vi "Test QR Code Memory Allocation.vi"(11 "Test Case In":refnum<class "02_FeatureDetection.lvclass">) -> (0 "error out":errorcluster, 3 "Test Case Out":refnum<class "02_FeatureDetection.lvclass">)   [LabVIEW 2020, in "test.lvlib" / "02_FeatureDetection.lvclass"]
uses:
  02_FeatureDetection.lvclass
  usr/local/natinst/LabVIEW-2024-64/vi.lib/Astemes/LUnit/Test Case.lvclass
  feature_detection/WeChat QR Code Detector/Detection.ctl
  common/Image Points Quad (Float).ctl
  common/Image Point (Float).ctl
  common/Image Size (Integer).ctl
  feature_detection/QR Code Encoder/Correction Levels.ctl
  feature_detection/QR Code Encoder/QR Code Encoder.lvclass/QR Code Encoder.ctl
  feature_detection/WeChat QR Code Detector/WeChat QR Code Detector.lvclass/WeChat QR Code Detector.ctl
  <vilib>/Astemes/LUnit/Test Case.lvclass/Test Case.ctl
  feature_detection/QR Code Encoder/Create (Structured Append).vi
  image/New Image (Greyscale Preallocated).vi
  image/New Image (Greyscale Array).vi
  image/Draw Image to Picture (Greyscale).vi
  feature_detection/WeChat QR Code Detector/Detect and Decode Multiple (Greyscale).vi
  feature_detection/QR Code Encoder/CreateCore.vi
  image/New Image (Greyscale Preallocated).vi/6598b9e0-8a08-46f5-91fd-ca1b87217137.vi
  image/Draw Image to Picture (Greyscale).vi/9ae995ca-ccda-485c-89ac-02736fde3e8e.vi
  feature_detection/WeChat QR Code Detector/Detect and Decode Multiple (Greyscale).vi/de44e2b3-a41c-416e-9770-09f180cbffa1.vi
  <vilib>/Astemes/LUnit/Append Pass Result.vi
  <vilib>/Astemes/LUnit/Append Fail Result.vi
  <vilib>/Astemes/LUnit/Run In UI.vi
  <vilib>/Utility/error.llb/Clear Errors.vi
  <vilib>/Utility/error.llb/Error Cluster From Error Code.vi
  feature_detection/QR Code Encoder/Encode (Structured Append).vi
  feature_detection/WeChat QR Code Detector/Create (Model Files Folder).vi
  feature_detection/QR Code Encoder/QR Code Encoder.lvclass
  feature_detection/WeChat QR Code Detector/WeChat QR Code Detector.lvclass
  image/image.lvlib
  <vilib>/Astemes/LUnit/Test Case.lvclass
  common/common.lvlib
panel:
  out "Picture":picture
  out "Array":cluster{"Detections":T1[]}[](array[cluster])
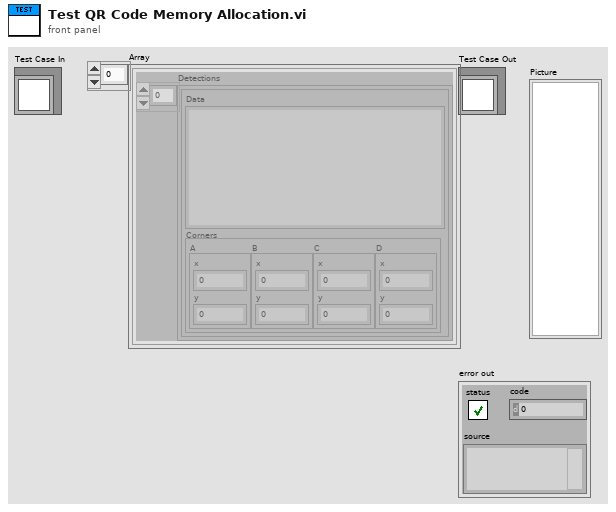
[diagram p1: front panel]
types:
  T1 = typedef "feature_detection.lvlib/WeChat QR Code Detector.lvclass/Detection.ctl" = cluster{"Data":string, "Corners":T2}
  T2 = typedef "common.lvlib/Image Points Quad (Float).ctl" = cluster{"A":T3, "B":T3, "C":T3, "D":T3}
  T3 = typedef "common.lvlib/Image Point (Float).ctl" = cluster{"x":dbl, "y":dbl}
  T4 = typedef "feature_detection.lvlib/QR Code Encoder.lvclass/Correction Levels.ctl" = enum16{"Level L", "Level M", "Level Q", "Level H"}
  T5 = typedef "common.lvlib/Image Size (Integer).ctl" = cluster{"Width":u16, "Height":u16}
  T6 = typedef "image.lvlib/Greyscale Image.ctl" = refnum<data-value>
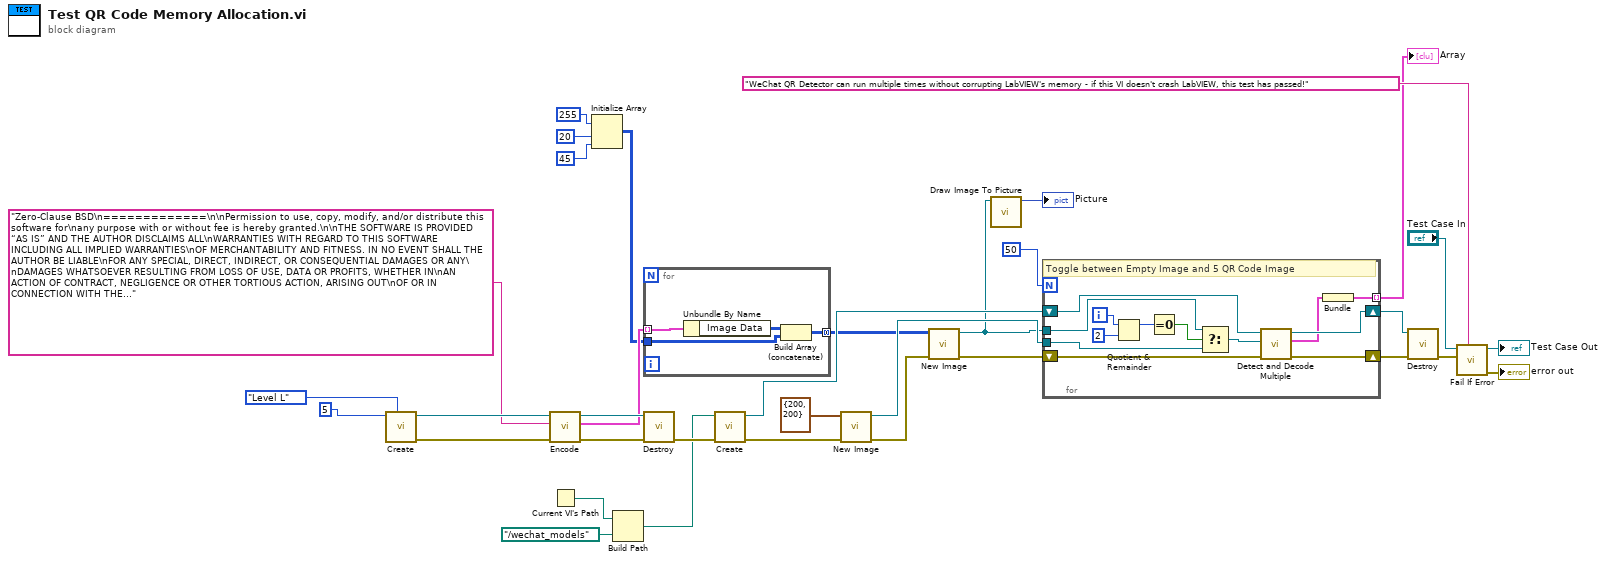
[diagram p0: block diagram]
diagram:
  n1 = call-poly "Create.vi"("Correction Level (Default: Level L)"=Correction_Levels."Level L", "Number of Structures"=u8 5) -> ("error out"=w18:errorcluster, "QR Code Encoder"=w20:refnum<class "QR Code Encoder.lvclass">)  [unwired: 8 in]
  n2 = call-poly "Encode.vi"("error in (no error)"=w18, "Data"="Zero-Clause BSD\n=============\n\nPermission to use, copy, modify, and/or distribute this software for\nany purpose with or without fee is hereby granted.\n\nTHE SOFTWARE IS PROVIDED “AS IS” AND THE AUTHOR DISCLAIMS ALL\nWARRANTIES WITH REGARD TO THIS SOFTWARE INCLUDING ALL IMPLIED WARRANTIES\nOF MERCHANTABILITY AND FITNESS. IN NO EVENT SHALL THE AUTHOR BE LIABLE\nFOR ANY SPECIAL, DIRECT, INDIRECT, OR CONSEQUENTIAL DAMAGES OR ANY\nDAMAGES WHATSOEVER RESULTING FROM LOSS OF USE, DATA OR PROFITS, WHETHER IN\nAN ACTION OF CONTRACT, NEGLIGENCE OR OTHER TORTIOUS ACTION, ARISING OUT\nOF OR IN CONNECTION WITH THE USE OR PERFORMANCE OF THIS SOFTWARE.", "QR Code Encoder in"=w20) -> ("error out"=w17:errorcluster, "QR Codes"=w9:cluster{"Image Data":u8[][]}[], "QR Code Encoder"=w19:refnum<class "QR Code Encoder.lvclass">)  [unwired: 6 in]
  n3 = Current VI's Path() -> (path=w3:path)
  n4 = Initialize Array(u8 255 ("element"), 20 ("dimension size"), 45 ("dimension size")) -> (w7:u8[][])
  n5 = Build Path(base path=w3, name or relative path=path "../wechat_models") -> (appended path=w2:path)
  n6 = for {
    tunnel: [w37] -> w14 mode=concatenating
    tunnel: w9 -> [w38] mode=indexing
    tunnel: w7 -> [w36]
    n7 = Unbundle By Name(w38) -> ("Image Data"=w35:u8[][])
    n8 = Build Array (concatenate)(w35, w36) -> (w37:u8[][])
  }
  n9 = call "Destroy.vi"("error in (no error)"=w17, "QR Code Encoder in"=w19) -> ("error out"=w15:errorcluster)  [unwired: 9 in]
  n10 = call-poly "Create.vi"("error in (no error)"=w15, "Model Files Directory"=w2) -> ("error out"=w30:errorcluster, "WeChat QR Code Detector"=w33:refnum<class "WeChat QR Code Detector.lvclass">)  [unwired: 8 in]
  n11 = call-poly "New Image.vi"("error in (no error)"=w30, "Preallocated Image Size (Default 0,0)"=T5 {"Width"=200, "Height"=200} ("Preallocated Image Size (Default: 0,0)")) -> ("error out"=w32:errorcluster, "Greyscale Image"=w31:T6)  [unwired: 8 in]
  n12 = call-poly "New Image.vi"("error in (no error)"=w32, "U8 Greyscale Data"=w14) -> ("error out"=w34:errorcluster, "Greyscale Image"=w13:T6)  [unwired: 8 in]
  n13 = call-poly "Draw Image To Picture.vi"("Greyscale Image Source in"=w13) -> ("Picture"=→"Picture":picture)  [unwired: 9 in, 1 out]
  n14 = for {
    N: 50 -> [_]
    tunnel: w13 -> [w45]
    tunnel: w31 -> [w44]
    shift-right: [w42] -> w29
    shift-left: w33 -> [w50]
    shift-right: [w41] -> w23
    shift-left: w34 -> [w51]
    tunnel: [w39] -> w21 mode=indexing
    i -> [w49]
    # "Toggle between Empty Image and 5 QR Code Image"
    n15 = Quotient & Remainder(x=w49, y=2) -> (x-y*floor(x/y)=w47:i32)  [unwired: 1 out]
    n16 = Equal To 0?(x=w47) -> (x = 0?=w46:bool)
    n17 = Select(t=w45, s=w46, f=w44) -> (s? t:f=w43:T6)
    n18 = call-poly "Detect and Decode Multiple.vi"("error in (no error)"=w51, "Greyscale Image in"=w43, "WeChat QR Code Detector in"=w50) -> ("error out"=w41:errorcluster, "Detections"=w40:T1[], "WeChat QR Code Detector"=w42:refnum<class "WeChat QR Code Detector.lvclass">)  [unwired: 6 in]
    n19 = Bundle("Detections"=w40) -> (w39:cluster{"Detections":T1[]})  [unwired: 1 in]
  }
  "Array" <- w21
  n20 = call "Destroy.vi"("error in (no error)"=w23, "WeChat QR Code Detector in"=w29) -> ("error out"=w22:errorcluster)  [unwired: 9 in]
  n21 = call <vilib>:"Fail If Error.vi"("Description"="WeChat QR Detector can run multiple times without corrupting LabVIEW's memory - if this VI doesn't crash LabVIEW, this test has passed!", "Assert error"=w22, "LUnit Test Case In"="Test Case In") -> ("error out"=→"error out":errorcluster, "LUnit Test Case Out"=→"Test Case Out":refnum<class "02_FeatureDetection.lvclass">)  [unwired: 7 in]
